vi "SpectAutoInt.vi"(3 "error in (no error)":errorcluster, 4 "Mode":enum16{"Stand Alone", "Runtime"}(ring), 5 "Integration Time":i32, 6 "SpectRef In":T3) -> (0 "error out":errorcluster, 1 "Saturated?":T2, 2 "SpectRef Out":T3)   [LabVIEW 2012]
uses:
  Controls/USB4000_Data.ctl
panel:
  out "Saturated? 2":bool
  out "output cluster":T1
  out "Array":dbl[](array[numeric])
  in  "appended array":T4(array[cluster])
  out "IntegrationTime":dbl
  out "Spect Raw":cluster{"all rows":dbl[], "all rows":dbl[]}[](graph)
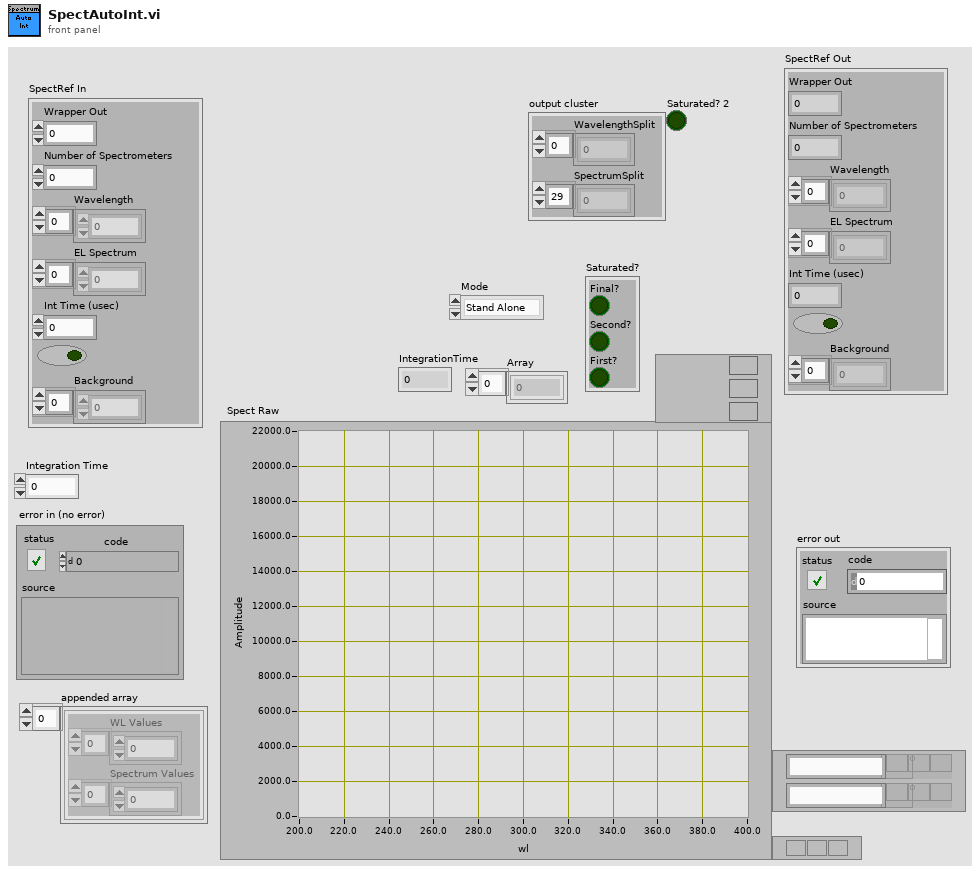
[diagram p1: front panel]
types:
  T1 = cluster{"WavelengthSplit":dbl[], "SpectrumSplit":dbl[]}
  T2 = cluster{"First?":bool, "Second?":bool, "Final?":bool}
  T3 = typedef "USB4000_Data.ctl" = cluster{"Wrapper Out":u32, "Number of Spectrometers":i32, "Wavelength":dbl[], "EL Spectrum":dbl[], "Int Time (usec)":i32, bool, "Background":dbl[]}
  T4 = cluster{"WL Values":dbl[], "Spectrum Values":dbl[]}[]
  T5 = cluster{"Final?":bool, "Second?":bool, "First?":bool}
  T6 = cluster{"WavelengthSplit":dbl[], "SpectrumSplit":dbl[]}[]
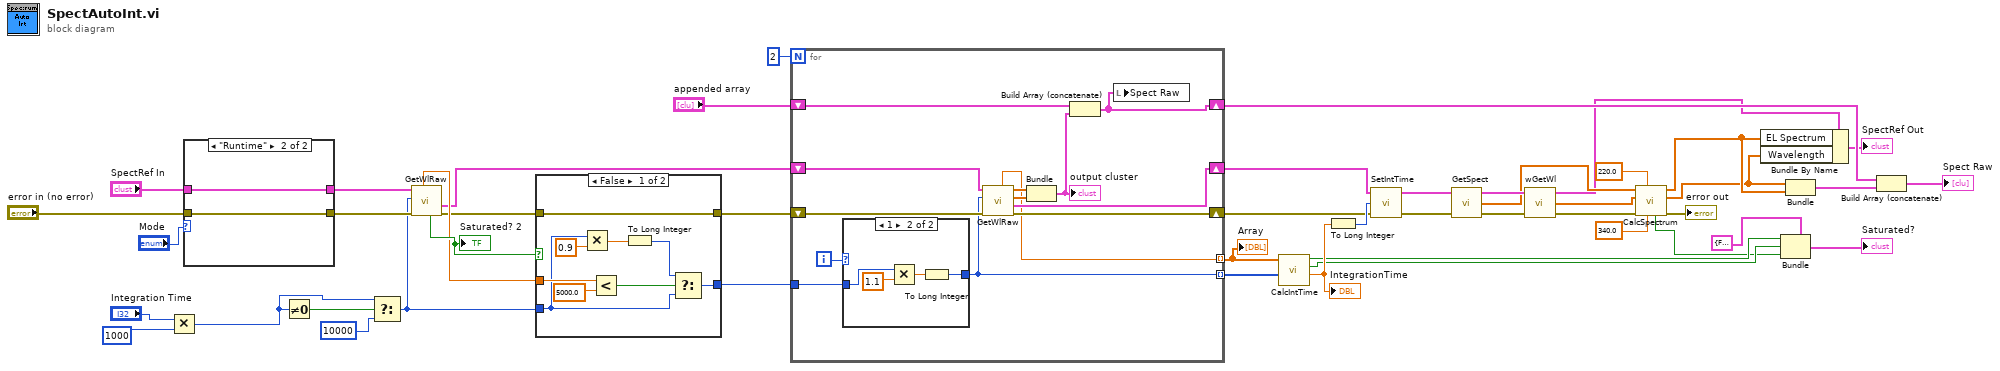
[diagram p0: block diagram]
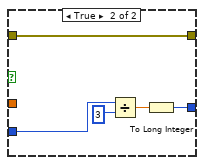
[diagram p2: hidden frame]
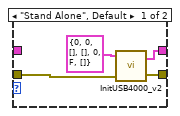
[diagram p3: hidden frame]
diagram:
  n1 = Multiply(x="Integration Time", y=1000) -> (x*y=w1:i32)
  n2 = case shown="\"Runtime\"" "Mode" {
    tunnel: [w50 w53] -> w12
    tunnel: [w49 w52] -> w11
    tunnel: "error in (no error)" -> [w48 w52]
    tunnel: "SpectRef In" -> [_ w53]
    frame "Stand Alone", Default {
      n3 = call "InitUSB4000_v2.vi"("error in (no error)"=w48, "USB4000 In"=T3 {"Wrapper Out"=0, "Number of Spectrometers"=0, "Wavelength"=[], "EL Spectrum"=[], "Int Time (usec)"=0, FALSE, "Background"=[]}) -> ("error out"=w49:errorcluster, "USB4000 Out"=w50:T3)  [unwired: 1 in]
    }
    frame "Runtime" {
    }
  }
  n4 = Not Equal To 0?(x=w1) -> (x != 0?=w24:bool)
  n5 = Select(t=w1, s=w24, f=10000 ("Integration Time")) -> (s? t:f=w9:i32)
  n6 = call "GetWlRaw.vi"("error in (no error)"=w11, "Integration Time"=w9, "SpectRef In"=w12) -> ("error out"=w4:errorcluster, "SpectRef Out"=w6:T3, "Saturated?"=w10:bool, "delta"=w7:dbl)  [unwired: 2 in, 3 out]
  "Saturated? 2" <- w10
  n7 = case shown="False" w10 {
    tunnel: w9 -> [w59 w67]
    tunnel: [w57 w64] -> w8
    tunnel: w7 -> [w62 _]
    tunnel: [w54 w63] -> w5
    tunnel: w4 -> [w54 w63]
    frame False {
      n8 = Multiply(x=w59, y=0.9) -> (x*y=w56:dbl)
      n9 = Less?(x=w62, y=5000.0) -> (x < y?=w60:bool)
      n10 = To Long Integer(number=w56) -> (32bit integer=w55:i32)
      n11 = Select(t=w55, s=w60, f=w59) -> (s? t:f=w57:i32)
    }
    frame True {
      n12 = Divide(x=w67, y=3) -> (x/y=w65:dbl)
      n13 = To Long Integer(number=w65) -> (32bit integer=w64:i32)
    }
  }
  n14 = for {
    N: 2 -> [_]
    shift-right: [w73] -> w35
    shift-left: w6 -> [w79]
    shift-right: [w70] -> w36
    shift-left: w5 -> [w78]
    shift-right: [w76] -> w34
    shift-left: "appended array" -> [w77]
    tunnel: w8 -> [w74]
    tunnel: [w69] -> w45 mode=indexing
    tunnel: [w68] -> w44 mode=indexing
    i -> [w75]
    n15 = case shown="1" w75 {
      tunnel: [w81 w82] -> w68
      tunnel: w74 -> [w81 w85]
      frame 0, Default {
      }
      frame 1 {
        n16 = Multiply(x=w85, y=1.1) -> (x*y=w83:dbl)
        n17 = To Long Integer(number=w83) -> (32bit integer=w82:i32)
      }
    }
    n18 = call "GetWlRaw.vi"("error in (no error)"=w78, "Integration Time"=w68, "SpectRef In"=w79) -> ("error out"=w70:errorcluster, "SpectRef Out"=w73:T3, "SpectrumSplit"=w71:dbl[], "WavelengthSplit"=w72:dbl[], "MaxSpectrum"=w69:dbl)  [unwired: 2 in, 2 out]
    n19 = Bundle("WavelengthSplit"=w72, "SpectrumSplit"=w71) -> (w80:T1)  [unwired: 1 in]
    "output cluster" <- w80
    n20 = Build Array (concatenate)(w77, w80) -> (w76:T6)
    n21 = local write "Spect Raw"(w76) -> ()
  }
  "Array" <- w45
  n22 = call "CalcIntTime.vi"("Int Time"=w44, "Array"=w45) -> ("IntegrationTime"=w38:dbl, "Saturated? 2"=w26:bool, "Saturated?"=w27:bool)  [unwired: 7 in]
  "IntegrationTime" <- w38
  n23 = To Long Integer(number=w38) -> (32bit integer=w37:i32)
  n24 = call "SetIntTime.vi"("error in"=w36, "Integration Time"=w37, "SpectRef In"=w35) -> ("error out"=w42:errorcluster, "SpectRef Out"=w40:T3)  [unwired: 1 in]
  n25 = call "GetSpect.vi"("error in (no error)"=w42, "SpectRef In"=w40) -> ("error out"=w43:errorcluster, "Spectrum Values"=w19:dbl[], "SpectRef Out"=w41:T3)  [unwired: 1 in]
  n26 = call "wGetWl.vi"("error in (no error)"=w43, "SpectRef In"=w41) -> ("error out"=w20:errorcluster, "WL Values"=w18:dbl[], "SpectRef Out"=w17:T3)  [unwired: 1 in]
  n27 = call "CalcSpectrum.vi"("WlStop"=340.0, "WlStart"=220.0, "error in (no error)"=w20, "Wavelength"=w18, "Spectrum"=w19) -> ("error out"=→"error out":errorcluster, "WavelengthSplit"=w13:dbl[], "SpectrumSplit"=w14:dbl[], "Saturated?"=w16:bool)  [unwired: 1 in, 2 out]
  n28 = Bundle By Name(cluster=w17, "EL Spectrum"=w14, "Wavelength"=w13) -> (→"SpectRef Out":T3)
  n29 = Bundle(cluster=T5 {"Final?"=FALSE, "Second?"=FALSE, "First?"=FALSE} ("Saturated?"), "Final?"=w27, "Second?"=w26, "First?"=w16) -> (→"Saturated?":T5)
  n30 = Bundle("WavelengthSplit"=w13, "SpectrumSplit"=w14) -> (w39:T1)  [unwired: 1 in]
  n31 = Build Array (concatenate)(w34, w39) -> (→"Spect Raw":T6)
